vi "spline position.vi"(10 "Data OUT in":T1={"Impulse Positions"=[], "No. Imp"=0, "Parameter Time Series"=[], "Parameter Impuls Series"=[], "Experiment Parameters"={"Freq"=0.0, "Vel"=0, "Acc"=0, "Stimulus"=""}, "Autosort File"=refnum, "Data File"={"Data Channels"=[], "Sample Rate"=0, "Channel List"=[]}, "Experiment data path"=path "", "Image data path"=path "", "LVS data path"=path "", "Raw copy path"=path "", "filename"="", "desaccading parameters"={"Tolerance"=0, "Acc Range"=0.0, "Sample Rate"=0, "Impulse Plane 2"=enum."Other", "Impulse dir"=FALSE}, "Experiment Parameters 2"={"Subject"="", "Strain"="", "Rotation plane"="", "Experimenter"="", "Trial"=0.0, "Time"=0.0}, "Excel"={"Excel._Application"=refnum, "Use Excel"=FALSE, "Worksheet SINE"=refnum, "Row SINE"=0, "Worksheet TRANS"=refnum, "Row TRANS"=0}, "Session Config File"=refnum, "Autosort Parameter Set"=0, "EMA Version"="", "desacc "={"Threshold 1 [Acc]"=0.0, "Threshold 2 [% of TH1]"=0, "tolerance"=0, "Search WD "=0.0, " always use TH2"=FALSE, "Range"=0.0, "Max time"=0.0, "Min time"=0.0, "Velocity Threshold"=0}, "Cycle Nr for Saccades"={"POS"=0, "NEG"=0}, "calibration name"="No file selected"} {"Parameter Time Series"."time offset" format="%.3f"; "Parameter Time Series"."Gain" format="%.1f"; "Parameter Time Series"."Offset" format="%.1f"; "Parameter Time Series"."List 1" items=["Motor-Pos", "Motor-Vel", "Lx Position-in-Head", "Ly Position-in-Head", "Lz Position-in-Head", "Lx Velocity-in-Head", "Ly Velocity-in-Head", "Lz Velocity-in-Head", "Ll Velocity-in-Head", "Lr Velocity-in-Head", "Lx Accel-in-Head", "Ly Accel-in-Head", "Lz Accel-in-Head", "Rx Position-in-Head", "Ry Position-in-Head", "Rz Position-in-Head", "Rx Velocity-in-Head", "Ry Velocity-in-Head", "Rz Velocity-in-Head", "Rl Velocity-in-Head", "Rr Velocity-in-Head", "Rx Accel-in-Head", "Ry Accel-in-Head", "Rz Accel-in-Head", "Global Trigger", "", "", ""]; "Parameter Impuls Series"."Gain" format="%.1f"; "Parameter Impuls Series"."Offset" format="%.1f"}, 11 "Digital in":refnum<vi>) -> (3 "Data OUT out":T1={"Impulse Positions"=[], "No. Imp"=0, "Parameter Time Series"=[], "Parameter Impuls Series"=[], "Experiment Parameters"={"Freq"=0.0, "Vel"=0, "Acc"=0, "Stimulus"=""}, "Autosort File"=refnum, "Data File"={"Data Channels"=[], "Sample Rate"=0, "Channel List"=[]}, "Experiment data path"=path "", "Image data path"=path "", "LVS data path"=path "", "Raw copy path"=path "", "filename"="", "desaccading parameters"={"Tolerance"=0, "Acc Range"=0.0, "Sample Rate"=0, "Impulse Plane 2"=enum."Other", "Impulse dir"=FALSE}, "Experiment Parameters 2"={"Subject"="", "Strain"="", "Rotation plane"="", "Experimenter"="", "Trial"=0.0, "Time"=0.0}, "Excel"={"Excel._Application"=refnum, "Use Excel"=FALSE, "Worksheet SINE"=refnum, "Row SINE"=0, "Worksheet TRANS"=refnum, "Row TRANS"=0}, "Session Config File"=refnum, "Autosort Parameter Set"=0, "EMA Version"="", "desacc "={"Threshold 1 [Acc]"=0.0, "Threshold 2 [% of TH1]"=0, "tolerance"=0, "Search WD "=0.0, " always use TH2"=FALSE, "Range"=0.0, "Max time"=0.0, "Min time"=0.0, "Velocity Threshold"=0}, "Cycle Nr for Saccades"={"POS"=0, "NEG"=0}, "calibration name"="No file selected"} {"Parameter Time Series"."time offset" format="%.3f"; "Parameter Time Series"."Gain" format="%.1f"; "Parameter Time Series"."Offset" format="%.1f"; "Parameter Time Series"."List 1" items=["Motor-Pos", "Motor-Vel", "Lx Position-in-Head", "Ly Position-in-Head", "Lz Position-in-Head", "Lx Velocity-in-Head", "Ly Velocity-in-Head", "Lz Velocity-in-Head", "Ll Velocity-in-Head", "Lr Velocity-in-Head", "Lx Accel-in-Head", "Ly Accel-in-Head", "Lz Accel-in-Head", "Rx Position-in-Head", "Ry Position-in-Head", "Rz Position-in-Head", "Rx Velocity-in-Head", "Ry Velocity-in-Head", "Rz Velocity-in-Head", "Rl Velocity-in-Head", "Rr Velocity-in-Head", "Rx Accel-in-Head", "Ry Accel-in-Head", "Rz Accel-in-Head", "Global Trigger", "", "", ""]; "Parameter Impuls Series"."Gain" format="%.1f"; "Parameter Impuls Series"."Offset" format="%.1f"})   [LabVIEW 2016]
uses:
  type-defs/TD_Statemachine-Data.ctl
  type-defs/TD_Time Series.ctl
  type-defs/TD_Impulse Parameter.ctl
  <vilib>/Analysis/3filter.llb/Savitzky-Golay Filter (DBL).vi
  <vilib>/Analysis/1siggen.llb/Ramp Pattern by Samples.vi
  comm/quaternion/quaternion.lvlib
  <vilib>/Analysis/NI_AALBase.lvlib
  <vilib>/Analysis/NI_AALPro.lvlib
  <vilib>/ptbypt/NI_PtbyPt.lvlib
  core.lvlib
panel:
  in  "Boolean":bool=TRUE
  in  "polynomial order":i32=3
  in  "side points":i32=6
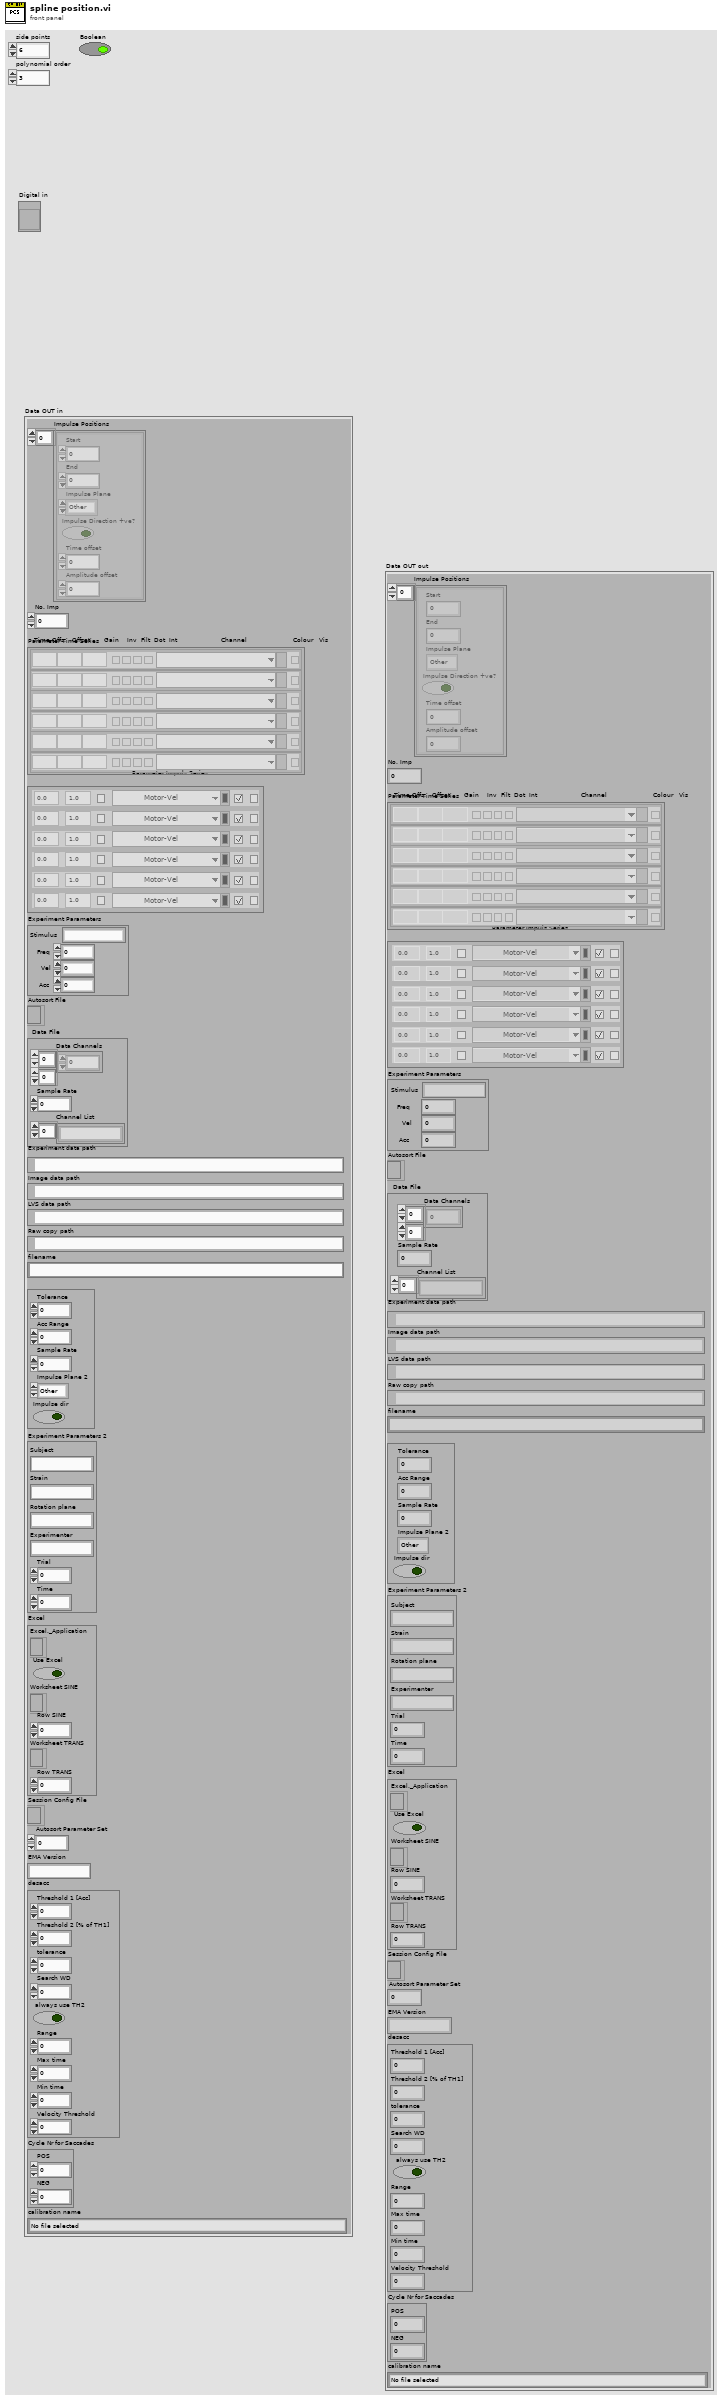
[diagram p1: front panel]
types:
  T1 = typedef "core.lvlib/TD_Statemachine-Data.ctl" = cluster{"Impulse Positions":cluster{"Start":i32, "End":i32, "Impulse Plane":enum16{"Other", "Yaw", "Pitch", "Roll", "LARP", "RALP"}, "Impulse Direction +ve?":bool, "Time offset":i32, "Amplitude offset":dbl}[], "No. Imp":i32, "Parameter Time Series":T2, "Parameter Impuls Series":T3, "Experiment Parameters":cluster{"Freq":dbl, "Vel":i32, "Acc":i32, "Stimulus":string}, "Autosort File":refnum<file>, "Data File":cluster{"Data Channels":dbl[][], "Sample Rate":i32, "Channel List":string[]}, "Experiment data path":path, "Image data path":path, "LVS data path":path, "Raw copy path":path, "filename":string, "desaccading parameters":cluster{"Tolerance":i32, "Acc Range":dbl, "Sample Rate":i32, "Impulse Plane 2":enum16{"Other", "Yaw", "Pitch", "Roll", "LARP", "RALP"}, "Impulse dir":bool}, "Experiment Parameters 2":cluster{"Subject":string, "Strain":string, "Rotation plane":string, "Experimenter":string, "Trial":dbl, "Time":dbl}, "Excel":cluster{"Excel._Application":refnum<k7>, "Use Excel":bool, "Worksheet SINE":refnum<k7>, "Row SINE":i32, "Worksheet TRANS":refnum<k7>, "Row TRANS":i32}, "Session Config File":refnum<file>, "Autosort Parameter Set":i32, "EMA Version":string, "desacc ":cluster{"Threshold 1 [Acc]":dbl, "Threshold 2 [% of TH1]":i32, "tolerance":i32, "Search WD ":dbl, " always use TH2":bool, "Range":dbl, "Max time":dbl, "Min time":dbl, "Velocity Threshold":i32}, "Cycle Nr for Saccades":cluster{"POS":i32, "NEG":i32}, "calibration name":string}
  T2 = typedef "core.lvlib/TD_Time Series.ctl" = cluster{"time offset":dbl, "Offset":dbl, "Gain":dbl, "inverse":bool, "filter data":bool, "dots":bool, "interpolate":bool, "List 1":u16, "Color Box":u32, "Boolean":bool}[]
  T3 = typedef "core.lvlib/TD_Impulse Parameter.ctl" = cluster{"Color":u32, "Visible":bool, "Channel":u16, "Invert":bool, "Desaccade":bool, "Offset":dbl, "Gain":dbl}[]
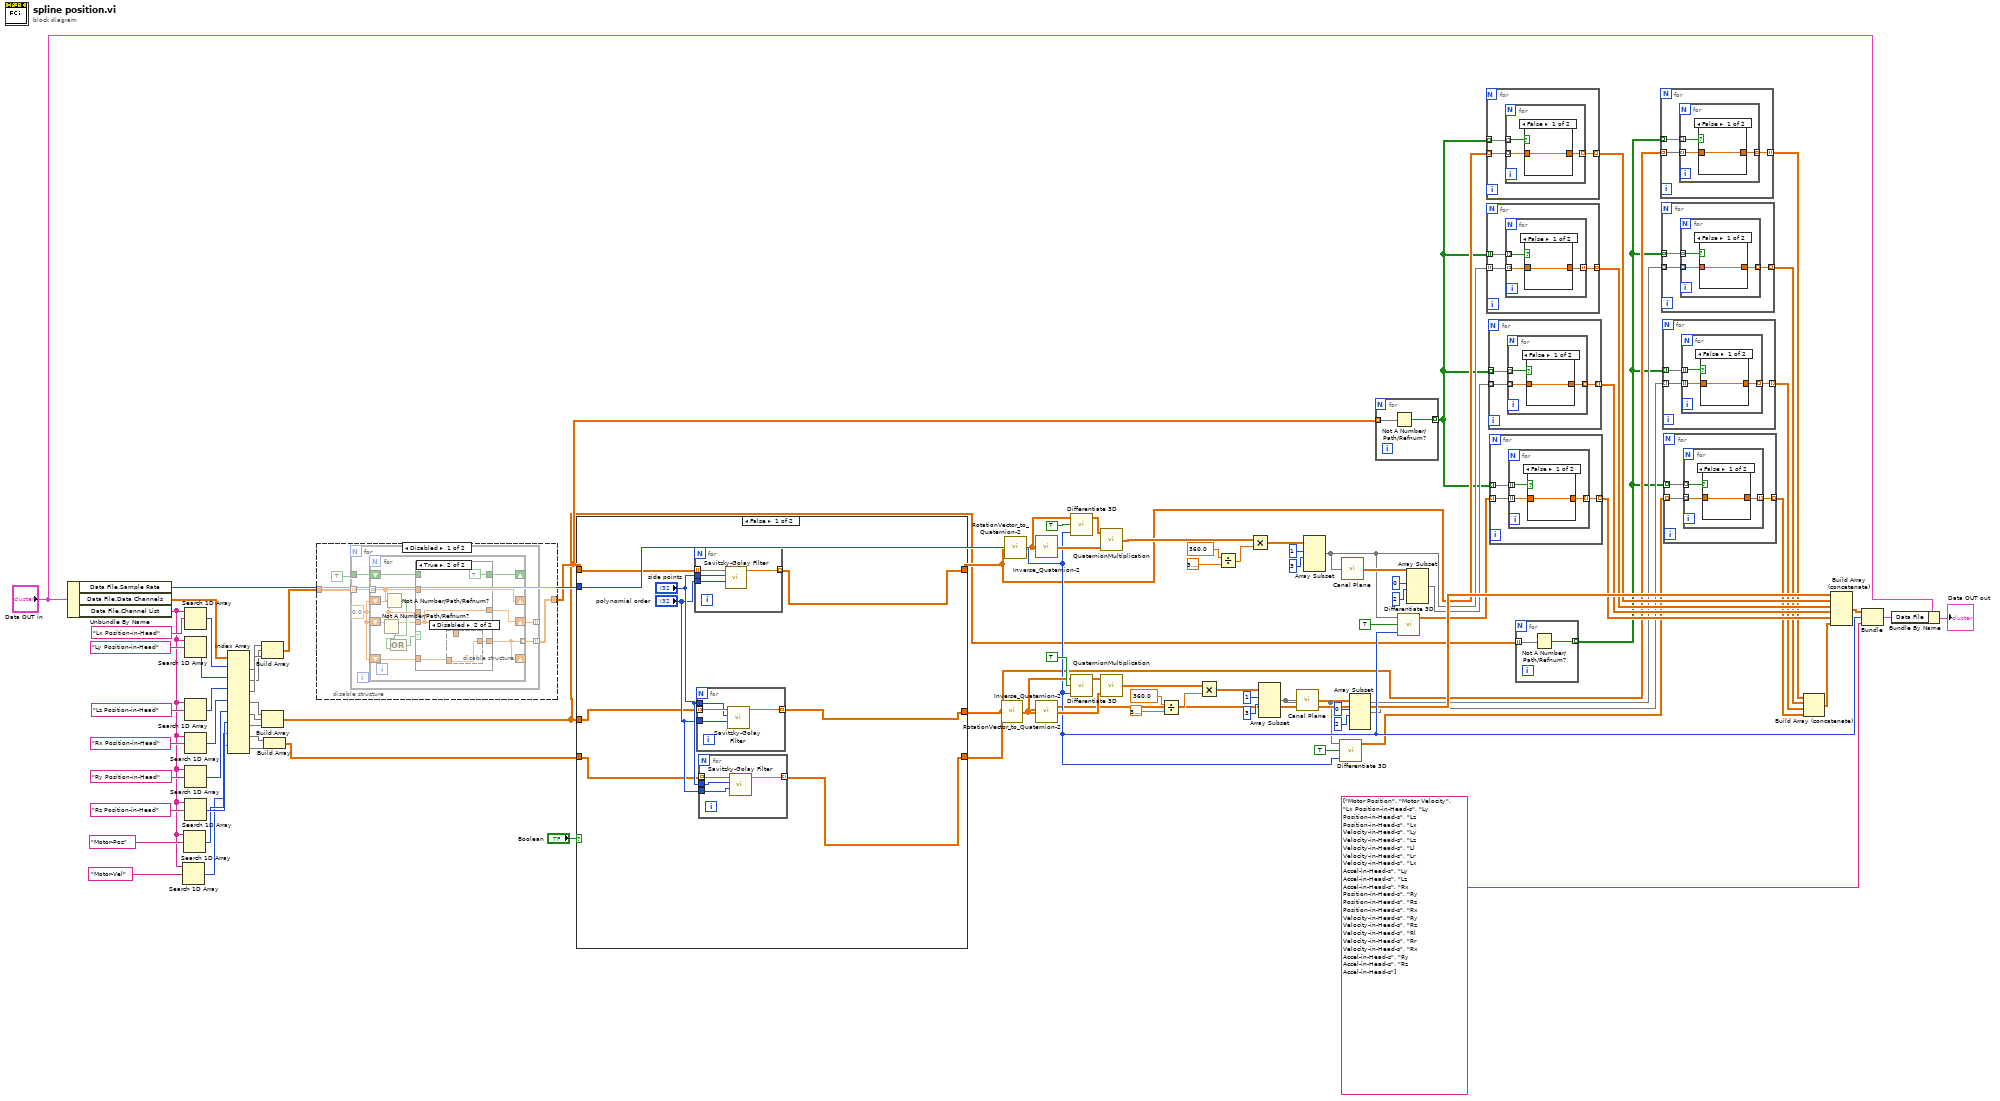
[diagram p0: block diagram]
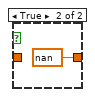
[diagram p2: hidden frame]
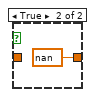
[diagram p3: hidden frame]
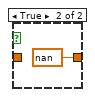
[diagram p4: hidden frame]
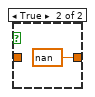
[diagram p5: hidden frame]
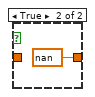
[diagram p6: hidden frame]
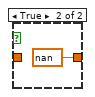
[diagram p7: hidden frame]
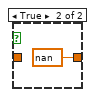
[diagram p8: hidden frame]
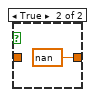
[diagram p9: hidden frame]
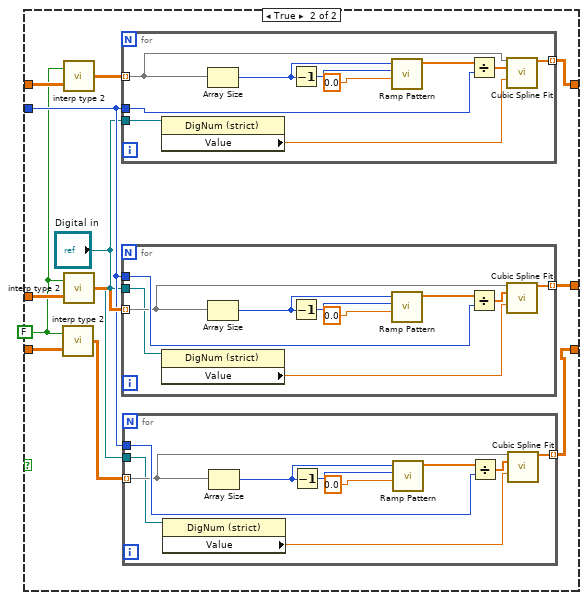
[diagram p10: hidden frame]
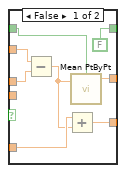
[diagram p11: hidden frame]
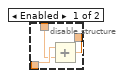
[diagram p12: hidden frame]
diagram:
  n1 = Unbundle By Name("Data OUT in") -> ("Data File.Sample Rate"=w25:i32, "Data File.Data Channels"=w56:dbl[][], "Data File.Channel List"=w30:string[])
  n2 = Search 1D Array(1D array=w30, element="Motor-Vel") -> (index of element=w29:i32)  [unwired: 1 in]
  n3 = Search 1D Array(1D array=w30, element="Motor-Pos") -> (index of element=w32:i32)  [unwired: 1 in]
  n4 = Search 1D Array(1D array=w30, element="Lx Position-in-Head") -> (index of element=w57:i32)  [unwired: 1 in]
  n5 = Search 1D Array(1D array=w30, element="Ly Position-in-Head") -> (index of element=w58:i32)  [unwired: 1 in]
  n6 = Search 1D Array(1D array=w30, element="Lz Position-in-Head") -> (index of element=w59:i32)  [unwired: 1 in]
  n7 = Search 1D Array(1D array=w30, element="Rx Position-in-Head") -> (index of element=w60:i32)  [unwired: 1 in]
  n8 = Search 1D Array(1D array=w30, element="Ry Position-in-Head") -> (index of element=w61:i32)  [unwired: 1 in]
  n9 = Search 1D Array(1D array=w30, element="Rz Position-in-Head") -> (index of element=w62:i32)  [unwired: 1 in]
  n10 = Index Array(array=w56, index (row) #1=w57, index (row) #2=w58, index (row) #3=w59, index (row) #4=w60, index (row) #5=w61, index (row) #6=w62, index (row) #7=w32, index (row) #8=w29) -> (element #1=w63:dbl[], element #2=w64:dbl[], element #3=w65:dbl[], element #4=w67:dbl[], element #5=w66:dbl[], element #6=w68:dbl[], element #7=w27:dbl[], element #8=w28:dbl[])  [unwired: 8 in]
  n11 = Build Array(w63, w64, w65) -> (w23:dbl[][])
  n12 = Build Array(w67, w66, w68) -> (w1:dbl[][])
  n13 = Build Array(w27, w28) -> (w26:dbl[][])
  n14 = disable-structure shown="Disabled" {
    disable-tunnel: w23 -> [w90 w123]
    disable-tunnel: [w89 w123] -> w11
    frame Disabled {
      n15 = for {
        tunnel: w90 -> [w95] mode=indexing
        tunnel: [w94] -> w89 mode=indexing
        tunnel: [w92] -> _ mode=indexing
        tunnel: TRUE -> [w91]
        w93 = 0.0
        n16 = for {
          tunnel: w95 -> [w105] mode=indexing
          shift-right: [w105] -> _
          shift-left: w93 -> [w106]
          tunnel: [w100] -> w94 mode=indexing
          shift-right: [w100] -> _
          shift-left: w93 -> [w101]
          shift-right: [w99] -> w92
          shift-left: w93 -> [w98]
          shift-right: [w96] -> _
          shift-left: w91 -> [w97]
          n17 = Not A Number/Path/Refnum?(number/path/refnum=w106) -> (NaN/Path/Refnum?=w103:bool)
          n18 = Not A Number/Path/Refnum?(number/path/refnum=w105) -> (NaN/Path/Refnum?=w104:bool)
          n19 = Compound Arithmetic op=OR(w104, w103) -> (w102:bool)
          n20 = case shown="True" w102 {
            tunnel: w105 -> [w114 _]
            tunnel: w106 -> [w113 _]
            tunnel: [w112 w117] -> w100
            tunnel: w101 -> [w111 w118]
            tunnel: [w109 w116] -> w99
            tunnel: w98 -> [_ w116]
            tunnel: w97 -> [w108 _]
            tunnel: [FALSE TRUE] -> w96
            frame False {
              n21 = Subtract(x=w114, y=w113) -> (x-y=w110:dbl)
              n22 = Add(x=w111, y=w110) -> (x+y=w112:dbl)
              n23 = call <vilib>:"Mean PtByPt.vi"("x"=w110, "initialize"=w108) -> ("mean"=w109:dbl)  [unwired: 2 in, 1 out]
            }
            frame True {
              n24 = disable-structure shown="Disabled" {
                disable-tunnel: w118 -> [w121 w122]
                disable-tunnel: [w120 w122] -> w117
                disable-tunnel: w116 -> [w119 _]
                frame Enabled {
                  n25 = Add(x=w121, y=w119) -> (x+y=w120:dbl)
                }
                frame Disabled {
                }
              }
            }
          }
        }
      }
    }
    frame Enabled {
    }
  }
  n26 = case shown="False" "Boolean" {
    tunnel: w1 -> [w128 w154]
    tunnel: [w126 w152] -> w4
    tunnel: w26 -> [w127 w151]
    tunnel: w25 -> [_ w149]
    tunnel: [w124 w147] -> w24
    tunnel: w11 -> [w129 w146]
    tunnel: [w125 w144] -> w14
    frame False {
      n27 = for {
        tunnel: w129 -> [w143] mode=indexing
        tunnel: [w142] -> w125 mode=indexing
        tunnel: "side points" -> [w141]
        tunnel: "polynomial order" -> [w140]
        n28 = call-poly <vilib>:"Savitzky-Golay Filter.vi"("polynomial order"=w140, "side points"=w141, "X"=w143) -> ("Filtered X"=w142:dbl[])  [unwired: 7 in, 1 out]
      }
      n29 = for {
        tunnel: w128 -> [w139] mode=indexing
        tunnel: [w138] -> w126 mode=indexing
        tunnel: "side points" -> [w137]
        tunnel: "polynomial order" -> [w136]
        n30 = call-poly <vilib>:"Savitzky-Golay Filter.vi"("polynomial order"=w136, "side points"=w137, "X"=w139) -> ("Filtered X"=w138:dbl[])  [unwired: 7 in, 1 out]
      }
      n31 = for {
        tunnel: w127 -> [w135] mode=indexing
        tunnel: [w134] -> w124 mode=indexing
        tunnel: "side points" -> [w133]
        tunnel: "polynomial order" -> [w132]
        n32 = call-poly <vilib>:"Savitzky-Golay Filter.vi"("polynomial order"=w132, "side points"=w133, "X"=w135) -> ("Filtered X"=w134:dbl[])  [unwired: 7 in, 1 out]
      }
    }
    frame True {
      w145 = FALSE ("Remove front and end")
      n33 = call "interp type 2.vi"("NaN"=w151, "Remove front and end"=w145) -> ("Interpolated"=w150:dbl[][])
      n34 = call "interp type 2.vi"("NaN"=w146, "Remove front and end"=w145) -> ("Interpolated"=w153:dbl[][])
      n35 = call "interp type 2.vi"("NaN"=w154, "Remove front and end"=w145) -> ("Interpolated"=w155:dbl[][])
      n36 = for {
        tunnel: w149 -> [w181]
        tunnel: w153 -> [w178] mode=indexing
        tunnel: [w179] -> w144 mode=indexing
        tunnel: "Digital in" -> [w176]
        n37 = property class="DigNum (strict)"(reference=w176) -> ("Value"=w177:dbl)  [unwired: 1 in, 2 out]
        n38 = Array Size(array=w178) -> (size(s)=w184:i32)
        n39 = Decrement(x=w184) -> (x-1=w183:i32)
        n40 = call-poly <vilib>:"Ramp Pattern.vi"("start"=0.0, "end"=w183, "samples"=w184) -> ("Ramp Pattern"=w182:dbl[])  [unwired: 7 in, 1 out]
        n41 = Divide(x=w182, y=w181) -> (x/y=w180:dbl[])
        n42 = call <vilib>:"Cubic Spline Fit.vi"("Y"=w178, "X"=w180, "balance parameter"=w177) -> ("Best Cubic Spline Fit"=w179:dbl[])  [unwired: 11 in, 1 out]
      }
      n43 = for {
        tunnel: w149 -> [w171]
        tunnel: w155 -> [w168] mode=indexing
        tunnel: [w169] -> w152 mode=indexing
        tunnel: "Digital in" -> [w166]
        n44 = property class="DigNum (strict)"(reference=w166) -> ("Value"=w167:dbl)  [unwired: 1 in, 2 out]
        n45 = Array Size(array=w168) -> (size(s)=w174:i32)
        n46 = Decrement(x=w174) -> (x-1=w173:i32)
        n47 = call-poly <vilib>:"Ramp Pattern.vi"("start"=0.0, "end"=w173, "samples"=w174) -> ("Ramp Pattern"=w172:dbl[])  [unwired: 7 in, 1 out]
        n48 = Divide(x=w172, y=w171) -> (x/y=w170:dbl[])
        n49 = call <vilib>:"Cubic Spline Fit.vi"("Y"=w168, "X"=w170, "balance parameter"=w167) -> ("Best Cubic Spline Fit"=w169:dbl[])  [unwired: 11 in, 1 out]
      }
      n50 = for {
        tunnel: w149 -> [w161]
        tunnel: w150 -> [w158] mode=indexing
        tunnel: [w159] -> w147 mode=indexing
        tunnel: "Digital in" -> [w156]
        n51 = property class="DigNum (strict)"(reference=w156) -> ("Value"=w157:dbl)  [unwired: 1 in, 2 out]
        n52 = Array Size(array=w158) -> (size(s)=w164:i32)
        n53 = Decrement(x=w164) -> (x-1=w163:i32)
        n54 = call-poly <vilib>:"Ramp Pattern.vi"("start"=0.0, "end"=w163, "samples"=w164) -> ("Ramp Pattern"=w162:dbl[])  [unwired: 7 in, 1 out]
        n55 = Divide(x=w162, y=w161) -> (x/y=w160:dbl[])
        n56 = call <vilib>:"Cubic Spline Fit.vi"("Y"=w158, "X"=w160, "balance parameter"=w157) -> ("Best Cubic Spline Fit"=w159:dbl[])  [unwired: 11 in, 1 out]
      }
    }
  }
  n57 = call "RotationVector_to_Quaternion-2.vi"("rotation vectors"=w4) -> ("quaternions"=w78:dbl[][])  [unwired: 4 in]
  n58 = call "RotationVector_to_Quaternion-2.vi"("rotation vectors"=w14) -> ("quaternions"=w22:dbl[][])  [unwired: 4 in]
  n59 = call "Inverse_Quaternion-2.vi"("quaternions"=w22) -> ("inverse quaternions"=w36:dbl[][])  [unwired: 4 in]
  n60 = call "Inverse_Quaternion-2.vi"("quaternions"=w78) -> ("inverse quaternions"=w70:dbl[][])  [unwired: 4 in]
  n61 = call "Differentiate 3D.vi"("Sample Rate 4"=w25, "Fixed Sample Rate"=TRUE, "Data (in)"=w22) -> ("Data (differentiated)"=w35:dbl[][])  [unwired: 2 in]
  n62 = call "Differentiate 3D.vi"("Sample Rate 4"=w25, "Fixed Sample Rate"=TRUE, "Data (in)"=w78) -> ("Data (differentiated)"=w69:dbl[][])  [unwired: 2 in]
  n63 = call "QuaternionMultiplication.vi"("quaternions B"=w36, "quaternions A"=w35) -> ("quaternions A x B"=w37:dbl[][])  [unwired: 3 in]
  n64 = call "QuaternionMultiplication.vi"("quaternions B"=w70, "quaternions A"=w69) -> ("quaternions A x B"=w71:dbl[][])  [unwired: 3 in]
  n65 = Divide(x=360.0, y=3.141592653589793) -> (x/y=w74:dbl)
  n66 = Multiply(x=w71, y=w74) -> (x*y=w83:dbl[][])
  n67 = Divide(x=360.0, y=3.141592653589793) -> (x/y=w40:dbl)
  n68 = Multiply(x=w37, y=w40) -> (x*y=w49:dbl[][])
  n69 = Array Subset(array=w83, index (row)=1 ("Array Index"), length (row)=3 ("Array Index")) -> (w6:dbl[][])  [unwired: 2 in]
  n70 = call "Canal Plane.vi"("Principal Planes"=w6) -> ("Canal Planes"=w75:dbl[][])
  n71 = Array Subset(array=w49, index (row)=1 ("Array Index"), length (row)=3 ("Array Index")) -> (w16:dbl[][])  [unwired: 2 in]
  n72 = call "Differentiate 3D.vi"("Sample Rate 4"=w25, "Fixed Sample Rate"=TRUE, "Data (in)"=w6) -> ("Data (differentiated)"=w10:dbl[][])  [unwired: 2 in]
  n73 = call "Canal Plane.vi"("Principal Planes"=w16) -> ("Canal Planes"=w41:dbl[][])
  n74 = Array Subset(array=w75, index (row)=0 ("Array Index"), length (row)=2 ("Array Index")) -> (w8:dbl[][])  [unwired: 2 in]
  n75 = for {
    tunnel: w11 -> [w187] mode=indexing
    tunnel: [w186] -> w12 mode=indexing
    n76 = Not A Number/Path/Refnum?(number/path/refnum=w187) -> (NaN/Path/Refnum?=w186:bool[])
  }
  n77 = call "Differentiate 3D.vi"("Sample Rate 4"=w25, "Fixed Sample Rate"=TRUE, "Data (in)"=w16) -> ("Data (differentiated)"=w20:dbl[][])  [unwired: 2 in]
  n78 = Array Subset(array=w41, index (row)=0 ("Array Index"), length (row)=2 ("Array Index")) -> (w18:dbl[][])  [unwired: 2 in]
  n79 = for {
    tunnel: w14 -> [w190] mode=indexing
    tunnel: [w189] -> w13 mode=indexing
    tunnel: w12 -> [w188] mode=indexing
    n80 = for {
      tunnel: w190 -> [w192] mode=indexing
      tunnel: [w193] -> w189 mode=indexing
      tunnel: w188 -> [w191] mode=indexing
      n81 = case shown="False" w191 {
        tunnel: [w194 nan] -> w193
        tunnel: w192 -> [w194 _]
        frame False {
        }
        frame True {
        }
      }
    }
  }
  n82 = for {
    tunnel: w16 -> [w198] mode=indexing
    tunnel: [w197] -> w15 mode=indexing
    tunnel: w12 -> [w196] mode=indexing
    n83 = for {
      tunnel: w198 -> [w200] mode=indexing
      tunnel: [w201] -> w197 mode=indexing
      tunnel: w196 -> [w199] mode=indexing
      n84 = case shown="False" w199 {
        tunnel: [w202 nan] -> w201
        tunnel: w200 -> [w202 _]
        frame False {
        }
        frame True {
        }
      }
    }
  }
  n85 = for {
    tunnel: w18 -> [w206] mode=indexing
    tunnel: [w205] -> w17 mode=indexing
    tunnel: w12 -> [w204] mode=indexing
    n86 = for {
      tunnel: w206 -> [w208] mode=indexing
      tunnel: [w209] -> w205 mode=indexing
      tunnel: w204 -> [w207] mode=indexing
      n87 = case shown="False" w207 {
        tunnel: [w210 nan] -> w209
        tunnel: w208 -> [w210 _]
        frame False {
        }
        frame True {
        }
      }
    }
  }
  n88 = for {
    tunnel: w12 -> [w214] mode=indexing
    tunnel: w20 -> [w213] mode=indexing
    tunnel: [w212] -> w19 mode=indexing
    n89 = for {
      tunnel: w214 -> [w217] mode=indexing
      tunnel: w213 -> [w215] mode=indexing
      tunnel: [w216] -> w212 mode=indexing
      n90 = case shown="False" w217 {
        tunnel: [w218 nan] -> w216
        tunnel: w215 -> [w218 _]
        frame False {
        }
        frame True {
        }
      }
    }
  }
  n91 = for {
    tunnel: w1 -> [w221] mode=indexing
    tunnel: [w220] -> w2 mode=indexing
    n92 = Not A Number/Path/Refnum?(number/path/refnum=w221) -> (NaN/Path/Refnum?=w220:bool[])
  }
  n93 = for {
    tunnel: w4 -> [w224] mode=indexing
    tunnel: [w223] -> w3 mode=indexing
    tunnel: w2 -> [w222] mode=indexing
    n94 = for {
      tunnel: w224 -> [w226] mode=indexing
      tunnel: [w227] -> w223 mode=indexing
      tunnel: w222 -> [w225] mode=indexing
      n95 = case shown="False" w225 {
        tunnel: [w228 nan] -> w227
        tunnel: w226 -> [w228 _]
        frame False {
        }
        frame True {
        }
      }
    }
  }
  n96 = for {
    tunnel: w6 -> [w232] mode=indexing
    tunnel: [w231] -> w5 mode=indexing
    tunnel: w2 -> [w230] mode=indexing
    n97 = for {
      tunnel: w232 -> [w234] mode=indexing
      tunnel: [w235] -> w231 mode=indexing
      tunnel: w230 -> [w233] mode=indexing
      n98 = case shown="False" w233 {
        tunnel: [w236 nan] -> w235
        tunnel: w234 -> [w236 _]
        frame False {
        }
        frame True {
        }
      }
    }
  }
  n99 = for {
    tunnel: w8 -> [w240] mode=indexing
    tunnel: [w239] -> w7 mode=indexing
    tunnel: w2 -> [w238] mode=indexing
    n100 = for {
      tunnel: w240 -> [w242] mode=indexing
      tunnel: [w243] -> w239 mode=indexing
      tunnel: w238 -> [w241] mode=indexing
      n101 = case shown="False" w241 {
        tunnel: [w244 nan] -> w243
        tunnel: w242 -> [w244 _]
        frame False {
        }
        frame True {
        }
      }
    }
  }
  n102 = for {
    tunnel: w2 -> [w248] mode=indexing
    tunnel: w10 -> [w247] mode=indexing
    tunnel: [w246] -> w9 mode=indexing
    n103 = for {
      tunnel: w248 -> [w251] mode=indexing
      tunnel: w247 -> [w249] mode=indexing
      tunnel: [w250] -> w246 mode=indexing
      n104 = case shown="False" w251 {
        tunnel: [w252 nan] -> w250
        tunnel: w249 -> [w252 _]
        frame False {
        }
        frame True {
        }
      }
    }
  }
  n105 = Build Array (concatenate)(w3, w5, w7, w9) -> (w84:dbl[][])
  n106 = Build Array (concatenate)(w24, w13, w15, w17, w19, w84) -> (w46:dbl[][])
  n107 = Bundle(w46, "Sample Rate"=w25, string[] ["Motor Position", "Motor Velocity", "Lx Position-in-Head-s", "Ly Position-in-Head-s", "Lz Position-in-Head-s", "Lx Velocity-in-Head-s", "Ly Velocity-in-Head-s", "Lz Velocity-in-Head-s", "Ll Velocity-in-Head-s", "Lr Velocity-in-Head-s", "Lx Accel-in-Head-s", "Ly Accel-in-Head-s", "Lz Accel-in-Head-s", "Rx Position-in-Head-s", "Ry Position-in-Head-s", "Rz Position-in-Head-s", "Rx Velocity-in-Head-s", "Ry Velocity-in-Head-s", "Rz Velocity-in-Head-s", "Rl Velocity-in-Head-s", "Rr Velocity-in-Head-s", "Rx Accel-in-Head-s", "Ry Accel-in-Head-s", "Rz Accel-in-Head-s"]) -> (w87:cluster{dbl[][], "Sample Rate":i32, string[]})  [unwired: 1 in]
  n108 = Bundle By Name(cluster="Data OUT in", "Data File"=w87) -> (→"Data OUT out":T1)
